vi "Check Command.vi"(7 "State":T1, 8 "error in (no error)":errorcluster, 11 "OBS in":refnum<class "OBS.lvclass">) -> (0 "error out":errorcluster, 3 "OBS out":refnum<class "OBS.lvclass">, 5 "Next State":T1)   [LabVIEW 2022 SP3, in "obs-websocket-lv.lvlib" / "OBS.lvclass"]
uses:
  OBS.lvclass
  State.ctl
  Command.ctl
  OBS.lvclass/OBS.ctl
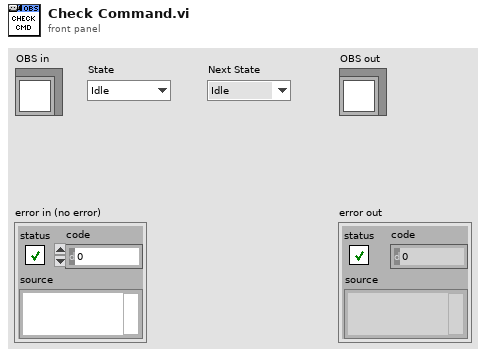
[diagram p1: front panel]
types:
  T1 = typedef "obs-websocket-lv.lvlib/OBS.lvclass/State.ctl" = enum16{"Idle", "Opening", "Open", "Closing", "Stopping"}
  T2 = typedef "obs-websocket-lv.lvlib/OBS.lvclass/Command.ctl" = enum16{"Open", "Close", "Stop"}
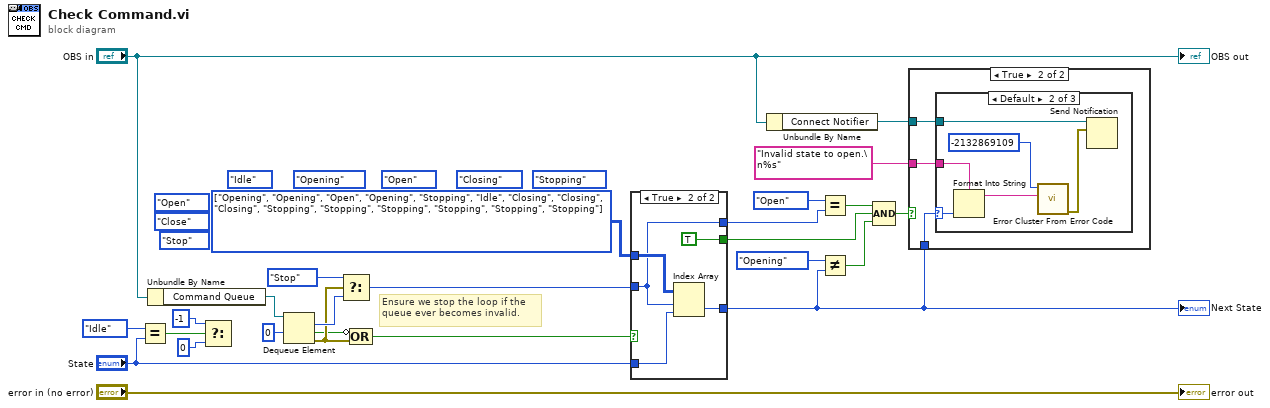
[diagram p0: block diagram]
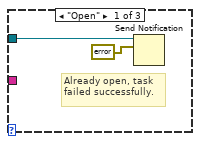
[diagram p3: hidden frame]
diagram:
  (unwired) State."Stopping" ("x")
  (unwired) State."Closing" ("x")
  (unwired) State."Open" ("x")
  (unwired) State."Opening" ("x")
  (unwired) State."Idle" ("x")
  (unwired) Command."Stop" ("Command")
  (unwired) Command."Close" ("Command")
  (unwired) Command."Open" ("Command")
  w19 = T1[][] [[enum."Opening", enum."Opening", enum."Open", enum."Opening", enum."Stopping"], [enum."Idle", enum."Closing", enum."Closing", enum."Closing", enum."Stopping"], [enum."Stopping", enum."Stopping", enum."Stopping", enum."Stopping", enum."Stopping"]] items=["Idle", "Opening", "Open", "Closing", "Stopping"]
  # "Ensure we stop the loop if the queue ever becomes invalid."
  n1 = Equal?(x=State."Idle", y="State") -> (x = y?=w23:bool)
  n2 = Unbundle By Name("OBS in") -> ("Command Queue"=w25:refnum<queue>)
  n3 = Select(t=-1, s=w23, f=0) -> ()  [unwired: 1 out]
  n4 = Dequeue Element(queue=w25, timeout in ms (-1)=0) -> (element=w7:T2, timed out?=w3:bool, error out=w4:errorcluster)  [unwired: 1 in, 1 out]
  n5 = Select(t=Command."Stop", s=w4, f=w7) -> (s? t:f=w6:T2)
  n6 = Compound Arithmetic op=OR(invert w3, w4) -> (w2:bool)
  n7 = case shown="True" w2 {
    tunnel: w6 -> [_ w28]
    tunnel: "State" -> [w27 w31]
    tunnel: w19 -> [_ w32]
    tunnel: [w27 w30] -> w11
    tunnel: [_ TRUE] -> w15
    tunnel: [_ w28] -> w17
    frame False {
    }
    frame True {
      n8 = Index Array(array=w32, index (row)=w28, index (col)=w31) -> (element=w30:T1)
    }
  }
  "Next State" <- w11
  n9 = Unbundle By Name("OBS in") -> ("Connect Notifier"=w9:refnum<notifier>)
  n10 = Equal?(x=Command."Open" ("y"), y=w17) -> (x = y?=w10:bool)
  n11 = Not Equal?(x=State."Opening", y=w11) -> (x != y?=w14:bool)
  n12 = Compound Arithmetic op=AND(w10, w15, w14) -> (w13:bool)
  n13 = case shown="True" w13 {
    tunnel: "Invalid state to open.\n%s" -> [_ w33]
    tunnel: w11 -> [_ w35]
    tunnel: w9 -> [_ w34]
    frame False {
    }
    frame True {
      n14 = case shown="Default" w35 {
        selector: w35 -> [_ w42 _]
        tunnel: w34 -> [w37 w39 _]
        tunnel: w33 -> [_ w43 _]
        frame "Open" {
          # "Already open, task failed successfully."
          n15 = Send Notification(notification=errorcluster {"status"=FALSE, "code"=0, "source"=""}, notifier=w37) -> ()  [unwired: 1 in, 2 out]
        }
        frame Default {
          n16 = Format Into String(format string=w43, w42) -> (resulting string=w41:string)  [unwired: 2 in, 1 out]
          n17 = call <vilib>:"Error Cluster From Error Code.vi"("error message (\"\")"=w41, "error code (0)"=-2132869109) -> ("error out"=w38:errorcluster)  [unwired: 7 in]
          n18 = Send Notification(notification=w38, notifier=w39) -> ()  [unwired: 1 in, 2 out]
        }
        frame "Opening" {
          # "Case not possible to reach and notification will be sent from Opening state code."
        }
      }
    }
  }
  "error out" <- "error in (no error)"
  "OBS out" <- "OBS in"
